vi "拉取压缩文件并解压缩.vi"(8 "error in (no error)":errorcluster, 10 "timeout (10000)":i32=300000, 11 "远端地址":string="/updatefiles/OneStation/V4/一体化微型水质监测站.zip") -> (0 "error out":errorcluster, 3 "文件路径":path)   [LabVIEW 2016, in "数据传输系统.lvlib" / "update.lvlib" / "http client.lvclass"]
uses:
  http client.lvclass
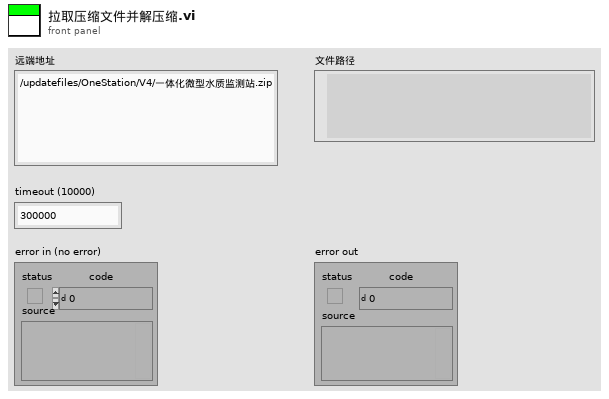
[diagram p1: front panel]
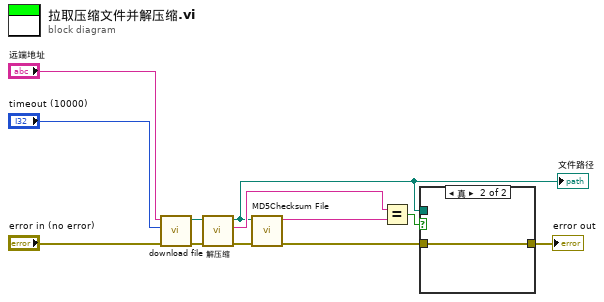
[diagram p0: block diagram]
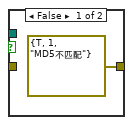
[diagram p2: hidden frame]
diagram:
  n1 = call "download file.vi"("error in (no error)"="error in (no error)", "timeout (10000)"="timeout (10000)", "远端地址"="远端地址") -> ("error out"=w10:errorcluster, "appended path"=w11:path)  [unwired: 7 in]
  n2 = call "解压缩.vi"("error in (no error)"=w10, "Zip file"=w11) -> ("error out"=w9:errorcluster, "MD5"=w4:string, "待校验的文件路径"=w2:path)  [unwired: 7 in]
  "文件路径" <- w2
  n3 = call <vilib>:"MD5Checksum File.vi"("error in (no error)"=w9, "Path"=w2) -> ("error out"=w7:errorcluster, "MD5 message-digest"=w3:string)  [unwired: 8 in]
  n4 = Equal?(x=w4, y=w3) -> (x = y?=w8:bool)
  n5 = case shown="真" w8 {
    tunnel: w2 -> [_ _]
    tunnel: w7 -> [_ w14]
    tunnel: [errorcluster {"status"=TRUE, "code"=1, "source"="MD5不匹配"} ("error out") w14] -> w5
    frame False {
    }
    frame True {
    }
  }
  "error out" <- w5
